vi "GetOperatorButtonPress.vi"(0 "GUI_Handler_Main in":refnum<class "GUI_Handler_Main.lvclass">, 5 "error in (no error)":errorcluster, 7 "Millisec timeout":u32=30000) -> (14 "GUI_Handler_Main out":refnum<class "GUI_Handler_Main.lvclass">, 16 "Operator_Aceept":bool, 17 "Operator_decline":bool, 18 "Timeout":bool, 19 "error out":errorcluster)   [LabVIEW 2017, in "GUI_Handler_Main.lvclass"]
uses:
  GUI_Handler_Main.lvclass
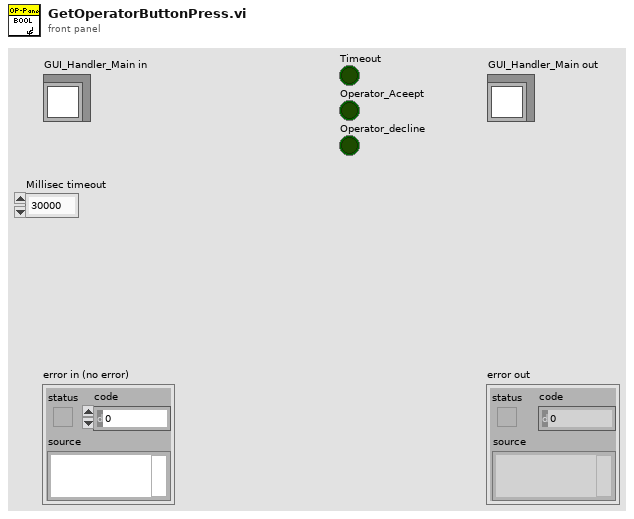
[diagram p1: front panel]
types:
  T1 = cluster{"Operator_Aceept":bool, "Operator_decline ":bool, "User message ":string}
  T2 = cluster{"Start Alt":refnum<vi>, "Stop":refnum<vi>, "Operatør beskeder":refnum<vi>}
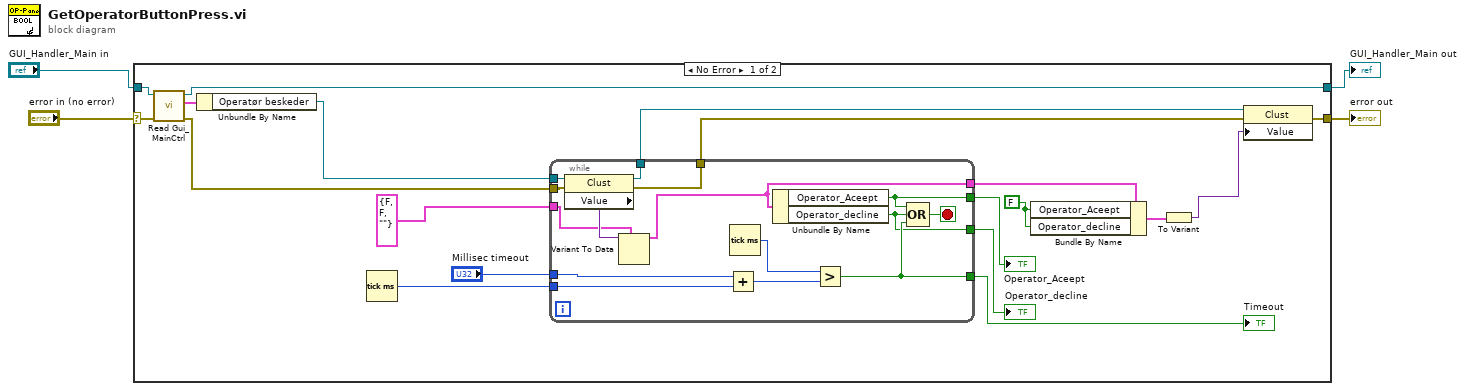
[diagram p0: block diagram]
diagram:
  n1 = case shown="No Error" "error in (no error)" {
    selector: "error in (no error)" -> [w19 w40]
    tunnel: [w20 w40] -> w3
    tunnel: [w22 w39] -> w1
    tunnel: "GUI_Handler_Main in" -> [w23 w39]
    frame No Error {
      w14 = FALSE ("Operator_Aceept")
      n2 = call-dynamic "Read Gui_MainCtrl.vi"("error in (no error)"=w19, "GUI_Handler_Main in"=w23) -> ("error out"=w9:errorcluster, "Gui_MainCtrl"=w21:T2, "GUI_Handler_Main out"=w22:refnum<class "GUI_Handler_Main.lvclass">)  [unwired: 7 in]
      n3 = Unbundle By Name(w21) -> ("Operatør beskeder"=w10:refnum<vi>)
      n4 = Tick Count (ms)() -> (millisecond timer value=w18:u32)
      n5 = while {
        tunnel: T1 {"Operator_Aceept"=FALSE, "Operator_decline "=FALSE, "User message "=""} ("Operatør beskeder") -> [w25]
        tunnel: w18 -> [w38]
        tunnel: "Millisec timeout" -> [w37]
        tunnel: [w33] -> w17
        tunnel: [w24] -> w13
        tunnel: [w32] -> w12
        tunnel: [w31] -> w11
        tunnel: w10 -> [w30]
        tunnel: w9 -> [w29]
        tunnel: [w28] -> w8
        tunnel: [w27] -> w7
        stop <- w34 stop-if-true
        n6 = property class="Clust"(reference=w30, error in=w29) -> (reference out=w28:refnum<vi>, error out=w27:errorcluster, "Value"=w26:variant)
        n7 = Variant To Data(type=w25, Variant=w26) -> (data=w24:T1)  [unwired: 1 in, 1 out]
        n8 = Add(x=w37, y=w38) -> (x+y=w36:u32)
        n9 = Tick Count (ms)() -> (millisecond timer value=w35:u32)
        n10 = Unbundle By Name(w24) -> ("Operator_Aceept"=w32:bool, "Operator_decline"=w31:bool)
        n11 = Greater?(x=w35, y=w36) -> (0:w33:bool)
        n12 = Compound Arithmetic op=OR(w32, w31, w33) -> (w34:bool)
      }
      "Timeout" <- w17
      "Operator_Aceept" <- w12
      "Operator_decline" <- w11
      n13 = Bundle By Name(cluster=w13, "Operator_Aceept"=w14, "Operator_decline"=w14) -> (w6:T1)
      n14 = To Variant(anything=w6) -> (Variant=w5:variant)
      n15 = property class="Clust"(reference=w8, error in=w7, "Value"=w5) -> (error out=w20:errorcluster)  [unwired: 1 out]
    }
    frame Error {
    }
  }
  "error out" <- w3
  "GUI_Handler_Main out" <- w1
